vi "Calibration Init.vi"(8 "error in (no error)":errorcluster) -> (0 "error out":errorcluster, 2 "Calibration Init Parameters Out":T1={"Readings Task"="All Readings", "Command Voltage Task"="Command Voltage", "samples per \nchannel"=30, "rate"=100.0, "Log File Path"=path "C:/Documents and Settings/mbletzin/Desktop/CalVolts.txt"})   [LabVIEW 2013]
uses:
  Calibration Init Parameters.ctl
panel:
  in  "Ok":bool
  in  "Calibration Init Parameters":T1={"Readings Task"="All Readings", "Command Voltage Task"="Command Voltage", "samples per \nchannel"=30, "rate"=100.0, "Log File Path"=path "C:/Documents and Settings/mbletzin/Desktop/CalVolts.txt"}
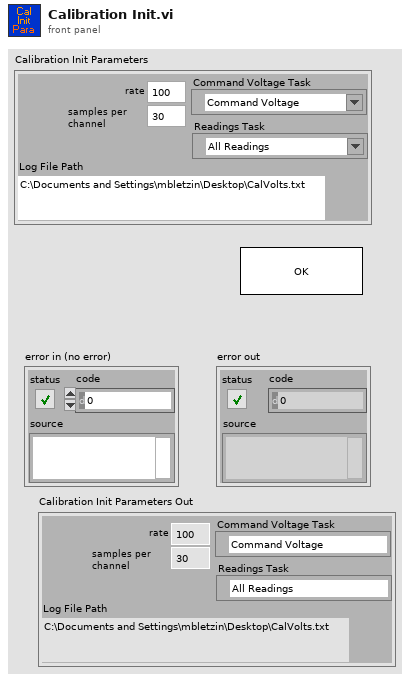
[diagram p1: front panel]
types:
  T1 = typedef "Calibration Init Parameters.ctl" = cluster{"Readings Task":refnum<k21>, "Command Voltage Task":refnum<k21>, "samples per \nchannel":i32, "rate":dbl, "Log File Path":path}
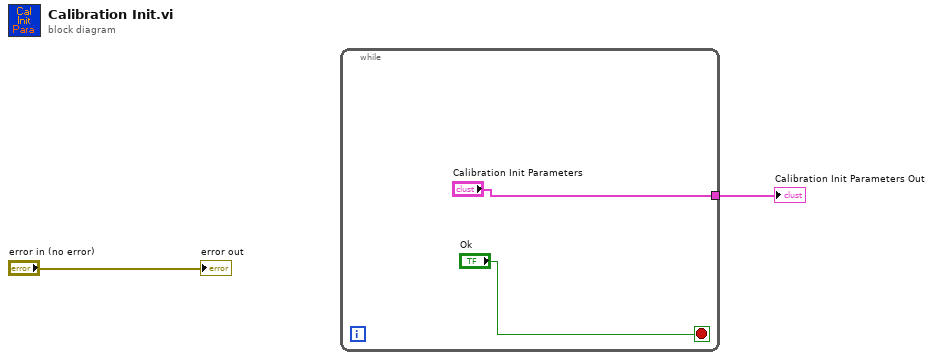
[diagram p0: block diagram]
diagram:
  n1 = while {
    tunnel: ["Calibration Init Parameters"] -> w2
    stop <- "Ok" stop-if-true
  }
  "Calibration Init Parameters Out" <- w2
  "error out" <- "error in (no error)"
